vi "Add Element in Available Sensors.vi"(8 "error in (no error)":errorcluster, 10 "Sensor In":refnum<class "Sensor.lvclass">, 11 "Vessel in":refnum<class "Vessel.lvclass">) -> (0 "error out":errorcluster, 3 "Vessel out":refnum<class "Vessel.lvclass">)   [LabVIEW 2014, in "Vessel.lvclass"]
uses:
  Vessel.lvclass
  Sensor/Sensor.lvclass
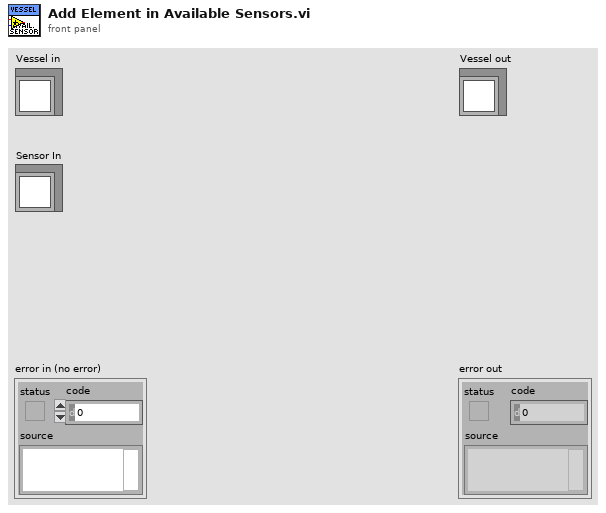
[diagram p1: front panel]
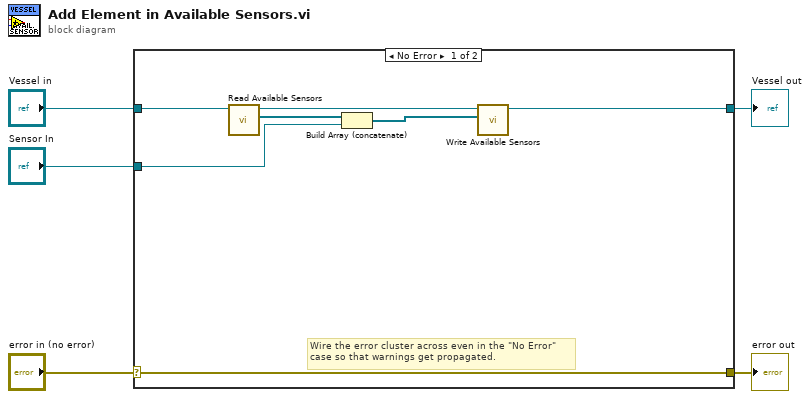
[diagram p0: block diagram]
diagram:
  n1 = case shown="No Error" "error in (no error)" {
    selector: "error in (no error)" -> [w12 w14]
    tunnel: [w12 w14] -> w4
    tunnel: [w6 w13] -> w2
    tunnel: "Vessel in" -> [w11 w13]
    tunnel: "Sensor In" -> [w9 _]
    frame No Error {
      # "Wire the error cluster across even in the \"No Error\"\ncase so that warnings get propagated."
      n2 = call "Read Available Sensors.vi"("Vessel in"=w11) -> ("Available Sensors"=w10:refnum<class "Sensor.lvclass">[], "Vessel out"=w8:refnum<class "Vessel.lvclass">)  [unwired: 8 in, 1 out]
      n3 = Build Array (concatenate)(w10, w9) -> (w7:refnum<class "Sensor.lvclass">[])
      n4 = call "Write Available Sensors.vi"("Available Sensors"=w7, "Vessel in"=w8) -> ("Vessel out"=w6:refnum<class "Vessel.lvclass">)  [unwired: 8 in, 1 out]
    }
    frame Error {
    }
  }
  "error out" <- w4
  "Vessel out" <- w2
